vi "CheckLostFrames.vi"(6 "Reset Lost Frames In":bool, 8 "Pause Acquisition in":bool, 9 "Last Image number":u32, 10 "Image Number":u32, 11 "LostFrames in":u32) -> (0 "Pause Acquisition out":bool, 1 "Last Image Number":u32, 3 "LostFrames out":u32, 4 "Reset Lost Frames Out":bool)   [LabVIEW 2013]
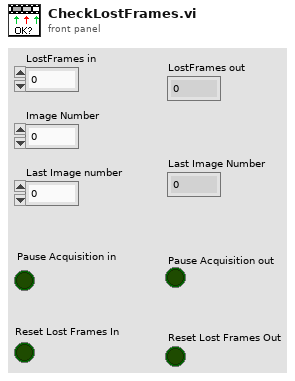
[diagram p1: front panel]
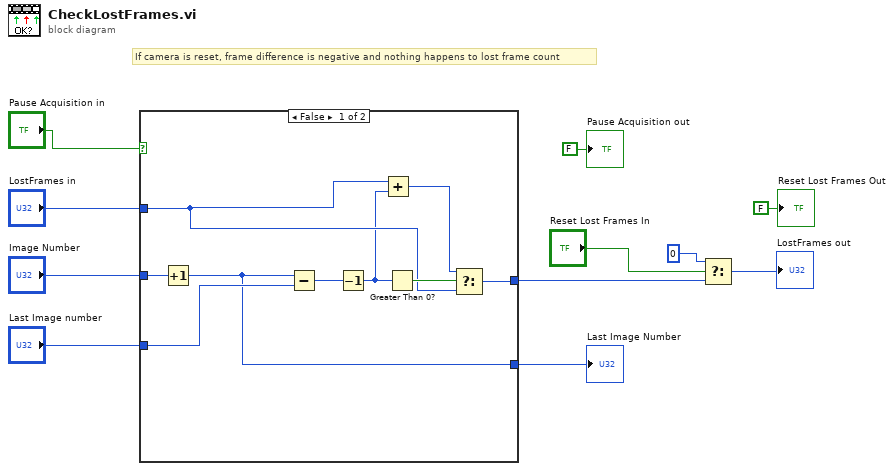
[diagram p0: block diagram]
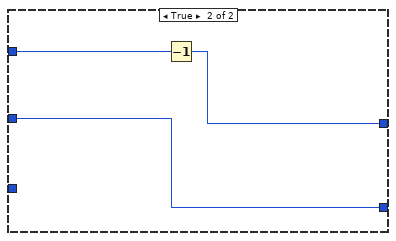
[diagram p2: hidden frame]
diagram:
  # "If camera is reset, frame difference is negative and nothing happens to lost frame count"
  n1 = case shown="False" "Pause Acquisition in" {
    tunnel: [w20 w21] -> w4
    tunnel: "Last Image number" -> [w17 _]
    tunnel: "Image Number" -> [w16 w23]
    tunnel: [w15 w23] -> w9
    tunnel: "LostFrames in" -> [w14 w22]
    frame False {
      n2 = Increment(x=w16) -> (x+1=w15:u32)
      n3 = Subtract(x=w15, y=w17) -> (x-y=w18:u32)
      n4 = Decrement(x=w18) -> (x-1=w13:u32)
      n5 = Add(x=w14, y=w13) -> (x+y=w12:u32)
      n6 = Greater Than 0?(x=w13) -> (x > 0?=w19:bool)
      n7 = Select(t=w12, s=w19, f=w14) -> (s? t:f=w20:u32)
    }
    frame True {
      n8 = Decrement(x=w22) -> (x-1=w21:u32)
    }
  }
  "Last Image Number" <- w9
  n9 = Select(t=u32 0, s="Reset Lost Frames In", f=w4) -> (s? t:f=→"LostFrames out":u32)
  "Pause Acquisition out" <- FALSE ("Pause Acquisition 2")
  "Reset Lost Frames Out" <- FALSE ("Reset Lost Frames Out")
